vi "Interface_Asset_Map Status.vi"(8 "error in (no error)":errorcluster, 11 "Load_Virtual in":refnum<class "Load_Virtual.lvclass">) -> (0 "error out":errorcluster, 3 "Load_Virtual out":refnum<class "Load_Virtual.lvclass">)   [LabVIEW 2015, in "Load_Virtual.lvclass"]
uses:
  Load_Virtual.lvclass
  Load.lvclass
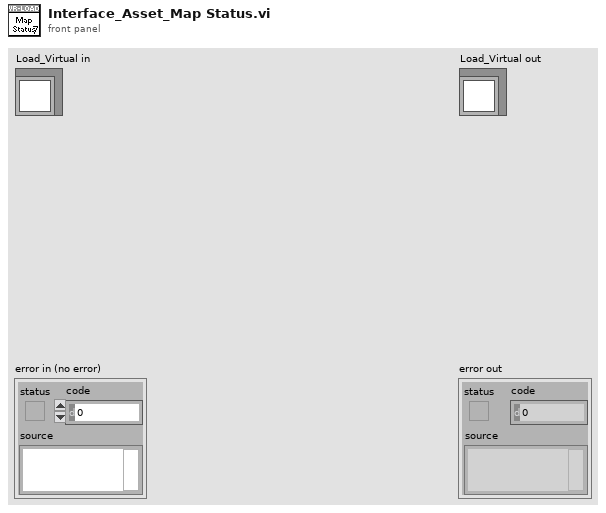
[diagram p1: front panel]
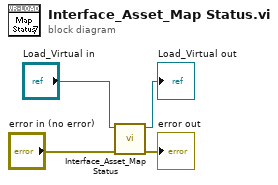
[diagram p0: block diagram]
diagram:
  n1 = call-parent "Interface_Asset_Map Status.vi"("error in (no error)"="error in (no error)", "Load in"="Load_Virtual in") -> ("error out"=→"error out":errorcluster, "Load out"=→"Load_Virtual out":refnum<class "Load_Virtual.lvclass">)  [unwired: 8 in]
